vi "TaskForVoiceControl_Cmd_Message.vi"(8 "error in (no error)":errorcluster caption="错误输入（无错误）", 10 "VoiceControl_Cmd_Cluster":T1, 11 "Actor in":refnum<class "ControlPanel.lvclass">) -> (0 "error out":errorcluster caption="错误输出", 3 "Actor out":refnum<class "ControlPanel.lvclass">)   [LabVIEW 2014, in "ControlPanel.lvlib" / "ControlPanel.lvclass"]
uses:
  ControlPanel.lvclass
  ControlPanel.lvclass/ControlPanel.ctl
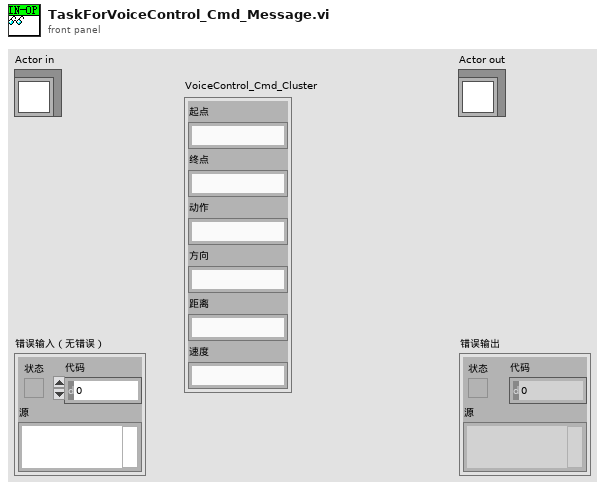
[diagram p1: front panel]
types:
  T1 = cluster{"起点":string, "终点":string, "动作":string, "方向":string, "距离":string, "速度":string}
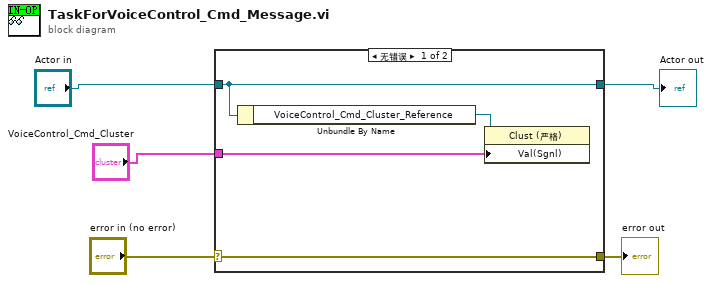
[diagram p0: block diagram]
diagram:
  n1 = case shown="无错误" "error in (no error)" {
    selector: "error in (no error)" -> [w9 w10]
    tunnel: [w9 w10] -> w4
    tunnel: [w8 w11] -> w1
    tunnel: "Actor in" -> [w8 w11]
    tunnel: "VoiceControl_Cmd_Cluster" -> [w6 _]
    frame No Error {
      n2 = Unbundle By Name(w8) -> ("VoiceControl_Cmd_Cluster_Reference"=w7:refnum<vi>)
      n3 = property class="Clust (严格)"(reference=w7, "Val(Sgnl)"=w6) -> ()  [unwired: 1 in, 2 out]
    }
    frame Error {
    }
  }
  "error out" <- w4
  "Actor out" <- w1
